vi "ABB extract array rows.vi"(9 "Row offset":i32, 10 "# rows":i32, 11 "Input array":string[][](array[string])) -> (1 "Next row":i32, 2 "First row":string[](array[string]), 3 "All rows":string[][](array[string]))   [LabVIEW 2017]
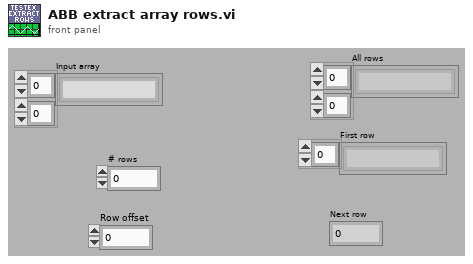
[diagram p1: front panel]
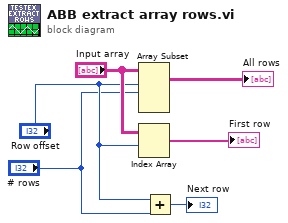
[diagram p0: block diagram]
diagram:
  n1 = Array Subset(array="Input array", index (row)="Row offset", length (row)="# rows") -> (→"All rows":string[][])  [unwired: 2 in]
  n2 = Index Array(array="Input array", index (row)="Row offset") -> (element=→"First row":string[])  [unwired: 1 in]
  n3 = Add(x="Row offset", y="# rows") -> (x+y=→"Next row":i32)
